vi "isSessionPresent.vi"(8 "error in":errorcluster, 10 "Client ID":string, 11 "MQTT_Base in":refnum<class "MQTT_Base.lvclass">) -> (0 "error out":errorcluster, 1 "Session Present":bool, 2 "Client ID dup":string, 3 "MQTT_Base out":refnum<class "MQTT_Base.lvclass">)   [LabVIEW 2013, in "MQTT Server.lvlib" / "MQTT_Base.lvclass"]
uses:
  MQTT_Base.lvclass
  Server/Session/Session State -- cluster.ctl
  Control Packets/SUBSCRIBE/Topic Subscription -- cluster.ctl
  Control Packets/ControlPacket/QualityOfService -- enum.ctl
  Control Packets/ControlPacket/Pending Transmission -- cluster.ctl
  Control Packets/ControlPacket/ControlPacket.lvclass
  Server/Session/Pending ACKs -- cluster.ctl
  Server/StoredSessions/StoredSessions.lvclass
  Server/Session/Session.lvclass
  Control Packets/SUBSCRIBE/SUBSCRIBE.lvclass
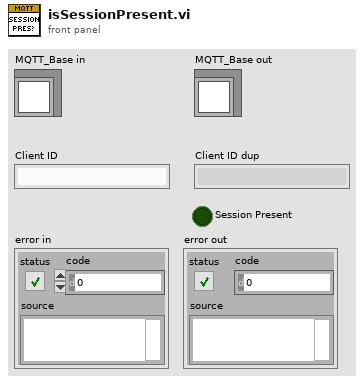
[diagram p1: front panel]
types:
  T1 = typedef "MQTT Server.lvlib/Session.lvclass/Session State -- cluster.ctl" = cluster{"CleanSession":bool, "Client ID":string, "Subscriptions":T2[], "Pending Transmissions":T4[], "Pending ACKs":T5[]}
  T2 = typedef "SUBSCRIBE.lvclass/Topic Subscription -- cluster.ctl" = cluster{"Topic Filter":string, "QoS":T3}
  T3 = typedef "ControlPacket.lvclass/QualityOfService -- enum.ctl" = enum16{"0 (At Most Once)", "1 (At Least Once)", "2 (Exactly Once)"}
  T4 = typedef "ControlPacket.lvclass/Pending Transmission -- cluster.ctl" = cluster{"Message":refnum<class "ControlPacket.lvclass">, "QoS":T3, "Tx-Rx":bool}
  T5 = typedef "MQTT Server.lvlib/Session.lvclass/Pending ACKs -- cluster.ctl" = cluster{"Message":refnum<class "ControlPacket.lvclass">, "[ACK]":refnum<notifier>[], "Packet Identifier":u16}
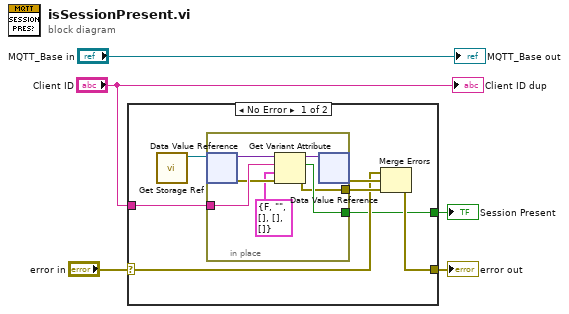
[diagram p0: block diagram]
diagram:
  n1 = case shown="No Error" "error in" {
    selector: "error in" -> [w8 w20]
    tunnel: [w7 w20] -> w4
    tunnel: "Client ID" -> [w11 _]
    tunnel: [w6 _] -> w3
    frame No Error {
      n2 = call "Get Storage Ref.vi"() -> ("Storage"=w12:refnum<data-value>)  [unwired: 11 in]
      n3 = in-place {
        in-place-border: w11 -> [w18]
        in-place-border: [w13] -> w10
        in-place-border: [w15] -> w6
        n4 = in-place-dvr #1(w12) -> (w19:variant, w16:errorcluster)
        n5 = Get Variant Attribute(Variant=w19, name=w18, default value (empty Variant)=T1 {"CleanSession"=FALSE, "Client ID"="", "Subscriptions"=[], "Pending Transmissions"=[], "Pending ACKs"=[]} ("Session State"), error in=w16) -> (duplicate Variant=w17:variant, found=w15:bool, error out=w13:errorcluster)  [unwired: 1 out]
        n6 = in-place-dvr #1(w17) -> (w9:errorcluster)  [unwired: 1 out]
      }
      n7 = Merge Errors(w8, w9, w10) -> (w7:errorcluster)
    }
    frame Error {
    }
  }
  "error out" <- w4
  "Session Present" <- w3
  "Client ID dup" <- "Client ID"
  "MQTT_Base out" <- "MQTT_Base in"
